vi "Init.vi"(7 "I2C #":T2=-1, 8 "error in (no error)":errorcluster, 10 "Session In":refnum<class "Session.lvclass">, 11 "Address":T1=39 format="%02x") -> (0 "error out":errorcluster, 2 "Session Out":refnum<class "Session.lvclass">, 3 "PCF8574 I2C LCD out":refnum<class "PCF8574 I2C LCD.lvclass">)   [LabVIEW 2020, in "CTI-Peripheral.lvlib" / "PCF8574 I2C LCD.lvclass"]
uses:
  PCF8574 I2C LCD.lvclass
  CTI/I2C Number.ctl
  CTI/Session/Session.lvclass
  CTI/I2C Address.ctl
  CTI/I2C Peripheral/I2C Peripheral.lvclass/I2C Peripheral.ctl
  PCF8574 I2C LCD.lvclass/PCF8574 I2C LCD.ctl
  CTI/I2C Peripheral/I2C Peripheral.lvclass
  CTI/CTI.lvlib
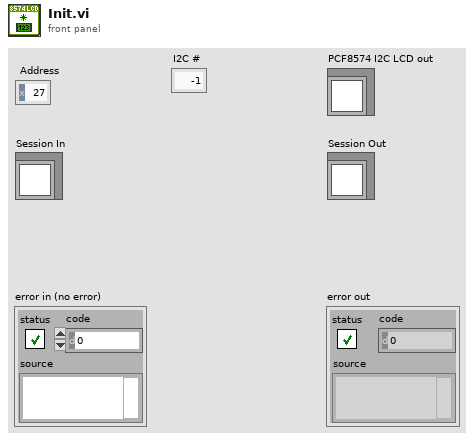
[diagram p1: front panel]
types:
  T1 = typedef "CTI.lvlib/I2C Address.ctl" = u8
  T2 = typedef "CTI.lvlib/I2C Number.ctl" = i8
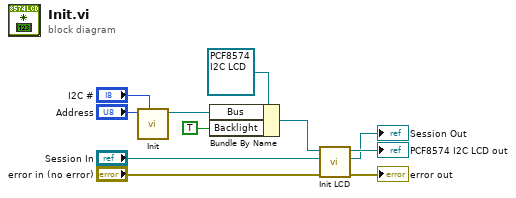
[diagram p0: block diagram]
diagram:
  n1 = call "Init.vi"("I2C"="I2C #", "Address"="Address") -> ("I2C Peripheral"=w7:refnum<class "I2C Peripheral.lvclass">)  [unwired: 8 in, 1 out]
  n2 = Bundle By Name(cluster=refnum<class "PCF8574 I2C LCD.lvclass"> refnum ("PCF8574 I2C LCD in"), "Bus"=w7, "Backlight"=TRUE) -> (w5:refnum<class "PCF8574 I2C LCD.lvclass">)
  n3 = call "Init LCD.vi"("error in (no error)"="error in (no error)", "Session In"="Session In", "PCF8574 I2C LCD in"=w5) -> ("error out"=→"error out":errorcluster, "Session Out"=→"Session Out":refnum<class "Session.lvclass">, "PCF8574 I2C LCD out"=→"PCF8574 I2C LCD out":refnum<class "PCF8574 I2C LCD.lvclass">)  [unwired: 6 in]
